vi "ABR-Plot Metrics.vi"(0 "Analysis":T1, 1 "Avg Mode":enum16{"Neural/CM", "ANOW"}(ring), 11 "error in (no error)":errorcluster, 12 "I-O":refnum<vi>) -> (15 "error out":errorcluster)   [LabVIEW 2020]
uses:
  TypeDefs/ABR-Analysis State.ctl
  Threshold Estimation VIs/ABR3-Threshold Estimation Result.ctl
  epl-vi-lib/Utility VIs/Graphics VIs/Graphics-Sort XY Graph (1D).vi
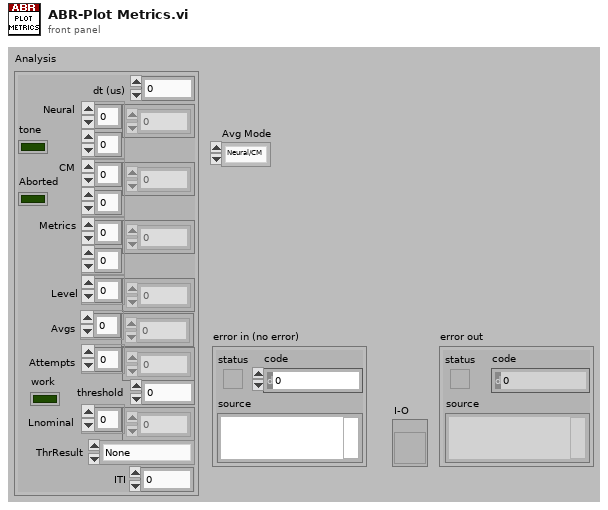
[diagram p1: front panel]
types:
  T1 = typedef "ABR-Analysis State.ctl" = cluster{"dt (us)":dbl, "Neural":dbl[][], "CM":dbl[][], "Metrics":dbl[][], "Level":dbl[], "Avgs":i32[], "Attempts":i32[], "Aborted":bool, "threshold":dbl, "Lnominal":dbl[], "tone":bool, "work":bool, "ThrResult":T2, "ITI":dbl}
  T2 = typedef "ABR3-Threshold Estimation Result.ctl" = enum16{"None", "Power", "Sigmoid", "Power (noisy)", "Suprathreshold", "Invalid"}
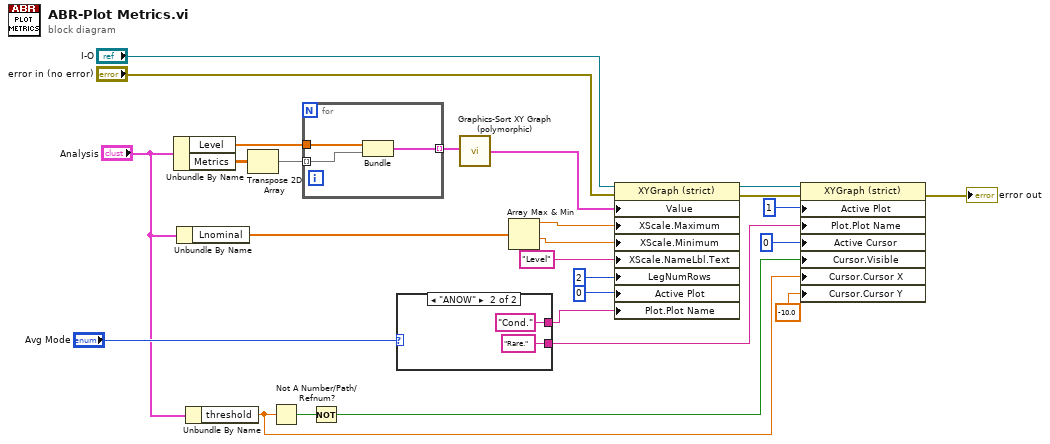
[diagram p0: block diagram]
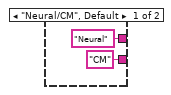
[diagram p2: hidden frame]
diagram:
  n1 = Unbundle By Name("Analysis") -> ("Level"=w25:dbl[], "Metrics"=w8:dbl[][])
  n2 = Unbundle By Name("Analysis") -> ("Lnominal"=w7:dbl[])
  n3 = Unbundle By Name("Analysis") -> ("threshold"=w2:dbl)
  n4 = Transpose 2D Array(2D array=w8) -> (transposed array=w21:dbl[][])
  n5 = Not A Number/Path/Refnum?(number/path/refnum=w2) -> (NaN/Path/Refnum?=w4:bool)
  n6 = for {
    tunnel: w25 -> [w28]
    tunnel: w21 -> [w27] mode=indexing
    tunnel: [w29] -> w10 mode=indexing
    n7 = Bundle("Level"=w28, w27) -> (w29:cluster{"Level":dbl[], dbl[]})  [unwired: 1 in]
  }
  n8 = Not(x=w4) -> (.not. x?=w3:bool)
  n9 = case shown="\"ANOW\"" "Avg Mode" {
    tunnel: ["Neural" ("Plot.Plot Name") "Cond." ("Plot.Plot Name")] -> w12
    tunnel: ["CM" ("Plot.Plot Name") "Rare." ("Plot.Plot Name")] -> w11
    frame "Neural/CM", Default {
    }
    frame "ANOW" {
    }
  }
  n10 = call-poly "Graphics-Sort XY Graph (polymorphic).vi"("graph"=w10) -> ("sorted graph"=w9:cluster{"x":dbl[], "y":dbl[]}[])  [unwired: 14 in]
  n11 = Array Max & Min(array=w7) -> (max value=w20:dbl, min value=w19:dbl)  [unwired: 2 out]
  n12 = property class="XYGraph (strict)"(reference="I-O", error in="error in (no error)", "Value"=w9, "XScale.Maximum"=w20, "XScale.Minimum"=w19, "XScale.NameLbl.Text"="Level" ("X Scale.Name Label.Text"), "LegNumRows"=u32 2 ("Legend:Number of Rows"), "Active Plot"=u32 0, "Plot.Plot Name"=w12) -> (reference out=w16:refnum<vi>, error out=w15:errorcluster)
  n13 = property class="XYGraph (strict)"(reference=w16, error in=w15, "Active Plot"=u32 1, "Plot.Plot Name"=w11, "Active Cursor"=u32 0, "Cursor.Visible"=w3, "Cursor.Cursor X"=w2, "Cursor.Cursor Y"=-10.0 ("Cursor.Cursor Position:Cursor Y")) -> (error out=→"error out":errorcluster)  [unwired: 1 out]
